vi "Parse RMC Sentence.vi"(8 "error in (no error)":errorcluster, 11 "RMC sentence":string) -> (0 "error out":errorcluster, 3 "RMC data":T1 {"type of fix"."mode" items=["", "Simulator", "Not Valid", "Estimated", "Differential", "Autonomous"]; "status"."value" items=["Void", "Active", ""]; "time of fix"."time" format="%^<%.3X\n%x>T"})   [LabVIEW 2011, in "u-blox 5 Series.lvlib"]
doc: "Returns data contained in an NMEA sentence. You must manually select the polymorphic instance to use."
uses:
  u-blox 5 Series.lvlib
  typedefs/RMC Data.ctl
  <vilib>/Utility/miscctls.llb/LVDateTimeRec.ctl
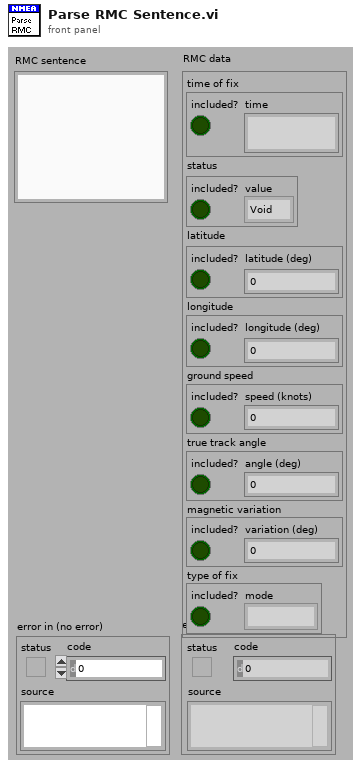
[diagram p1: front panel]
types:
  T1 = typedef "u-blox 5 Series.lvlib/RMC Data.ctl" = cluster{"time of fix":cluster{"included?":bool, "time":timestamp}, "status":cluster{"included?":bool, "value":u16}, "latitude":cluster{"included?":bool, "latitude (deg)":dbl}, "longitude":cluster{"included?":bool, "longitude (deg)":dbl}, "ground speed":cluster{"included?":bool, "speed (knots)":dbl}, "true track angle":cluster{"included?":bool, "angle (deg)":dbl}, "magnetic variation":cluster{"included?":bool, "variation (deg)":dbl}, "type of fix":cluster{"included?":bool, "mode":u16}}
  T2 = typedef "LVDateTimeRec.ctl" = cluster{"fractional second":dbl, "second":i32, "minute":i32, "hour":i32, "day of month":i32, "month":i32, "year":i32, "day of week":i32, "day of year":i32, "DST":i32}
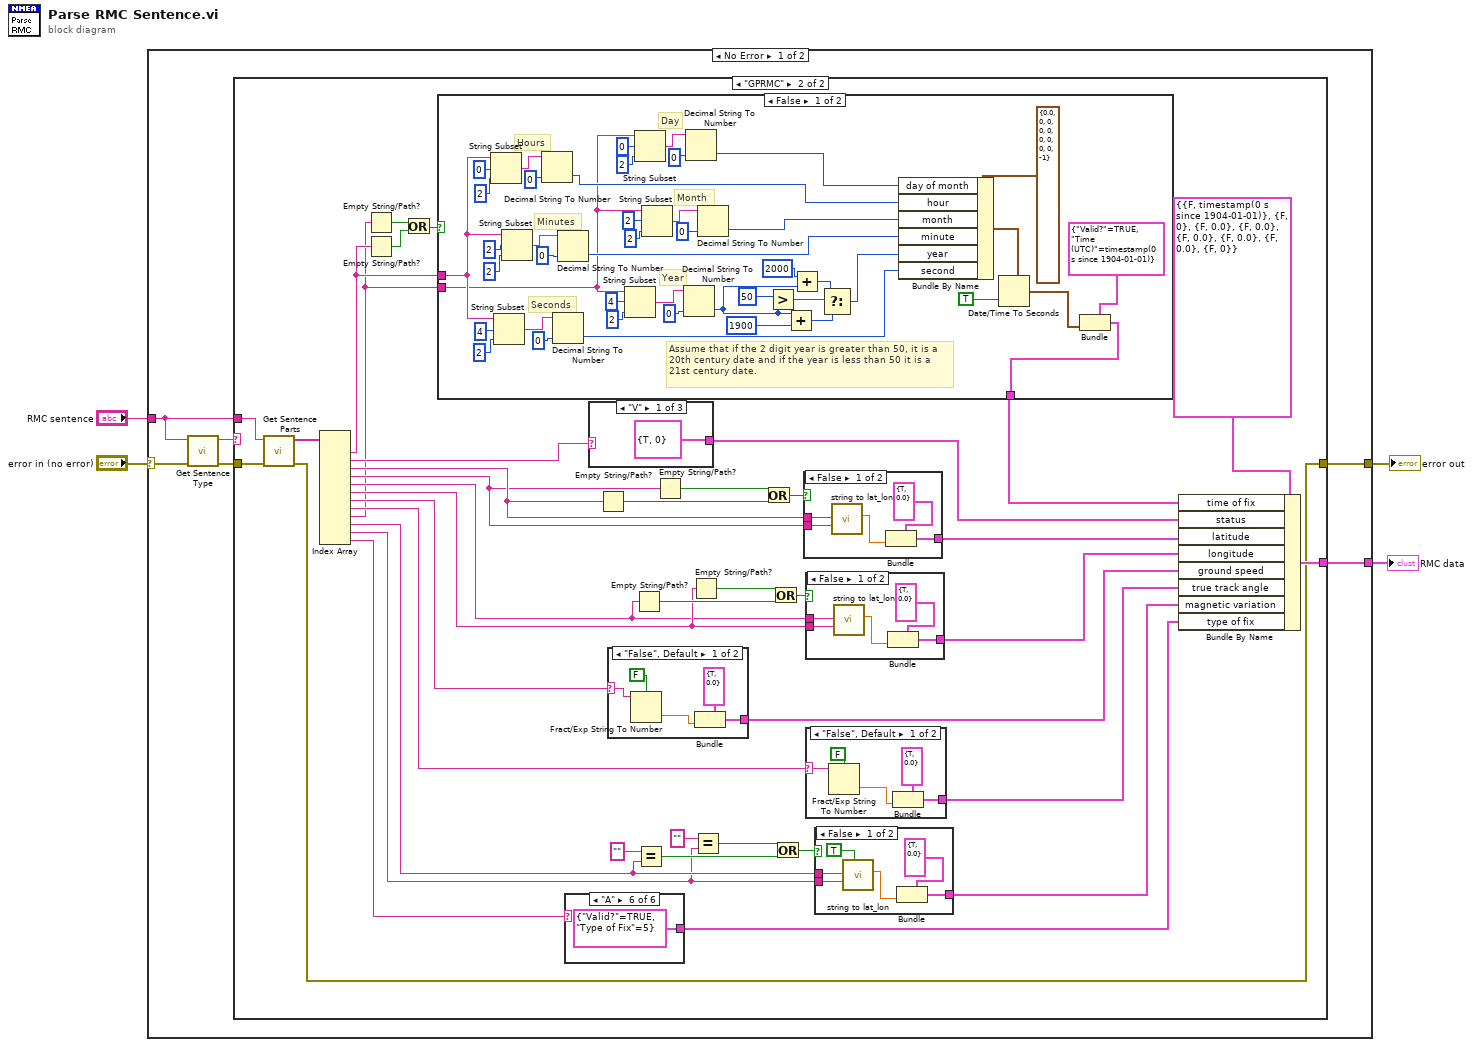
[diagram p0: block diagram]
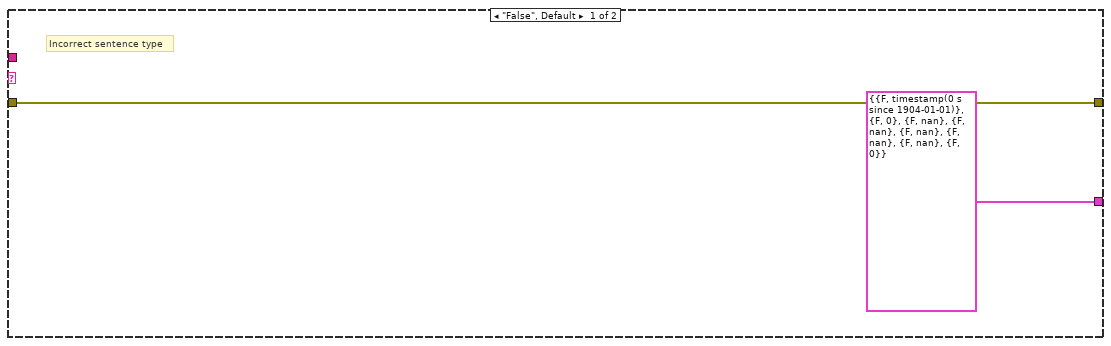
[diagram p2: hidden frame]
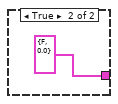
[diagram p3: hidden frame]
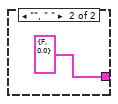
[diagram p4: hidden frame]
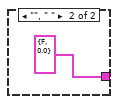
[diagram p5: hidden frame]
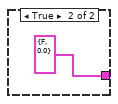
[diagram p6: hidden frame]
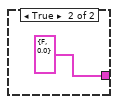
[diagram p7: hidden frame]
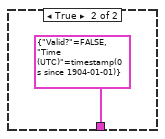
[diagram p8: hidden frame]
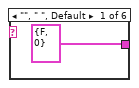
[diagram p9: hidden frame]
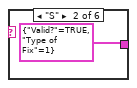
[diagram p10: hidden frame]
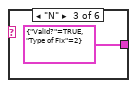
[diagram p11: hidden frame]
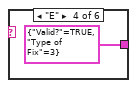
[diagram p12: hidden frame]
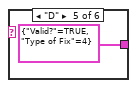
[diagram p13: hidden frame]
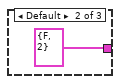
[diagram p14: hidden frame]
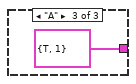
[diagram p15: hidden frame]
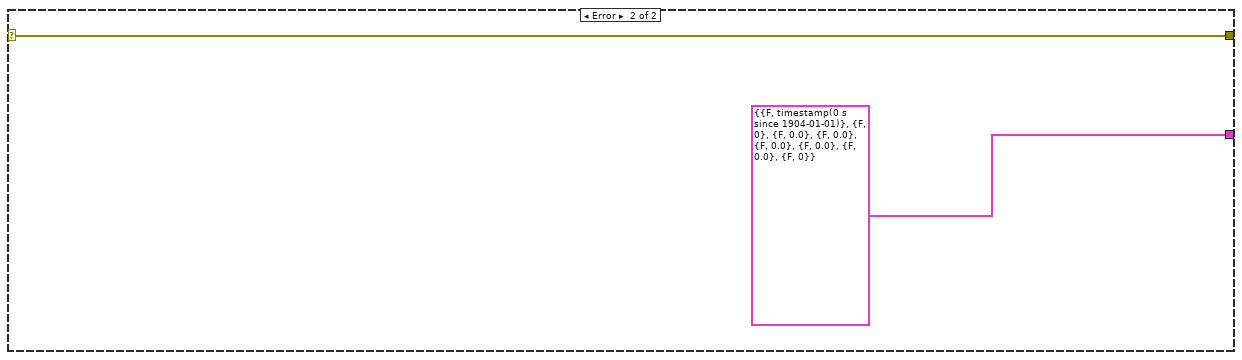
[diagram p16: hidden frame]
diagram:
  n1 = case shown="No Error" "error in (no error)" {
    selector: "error in (no error)" -> [w8 w140]
    tunnel: [w9 w140] -> w2
    tunnel: [w10 T1 {"time of fix"={"included?"=FALSE, "time"=timestamp(0 s since 1904-01-01)}, "status"={"included?"=FALSE, "value"=0}, "latitude"={"included?"=FALSE, "latitude (deg)"=0.0}, "longitude"={"included?"=FALSE, "longitude (deg)"=0.0}, "ground speed"={"included?"=FALSE, "speed (knots)"=0.0}, "true track angle"={"included?"=FALSE, "angle (deg)"=0.0}, "magnetic variation"={"included?"=FALSE, "variation (deg)"=0.0}, "type of fix"={"included?"=FALSE, "mode"=0}} ("RMC Data")] -> w1
    tunnel: "RMC sentence" -> [w6 _]
    frame No Error {
      n2 = call "Get Sentence Type.vi"("error in (no error)"=w8, "sentence"=w6) -> ("error out"=w7:errorcluster, "sentence type"=w5:string)  [unwired: 1 in, 7 out]
      n3 = case shown="\"GPRMC\"" w5 {
        tunnel: w6 -> [_ w16]
        tunnel: w7 -> [w11 w52]
        tunnel: [T1 {"time of fix"={"included?"=FALSE, "time"=timestamp(0 s since 1904-01-01)}, "status"={"included?"=FALSE, "value"=0}, "latitude"={"included?"=FALSE, "latitude (deg)"=nan}, "longitude"={"included?"=FALSE, "longitude (deg)"=nan}, "ground speed"={"included?"=FALSE, "speed (knots)"=nan}, "true track angle"={"included?"=FALSE, "angle (deg)"=nan}, "magnetic variation"={"included?"=FALSE, "variation (deg)"=nan}, "type of fix"={"included?"=FALSE, "mode"=0}} ("RMC Data") w51] -> w10
        tunnel: [w11 w14] -> w9
        frame "False", Default {
          # "Incorrect sentence type"
        }
        frame "GPRMC" {
          n4 = call "Get Sentence Parts.vi"("error in (no error)"=w52, "sentence"=w16) -> ("error out"=w14:errorcluster, "sentence data"=w15:string[])  [unwired: 1 in, 7 out]
          n5 = Index Array(array=w15) -> (element #1=w44:string, element #2=w49:string, element #3=w40:string, element #4=w39:string, element #5=w30:string, element #6=w31:string, element #7=w29:string, element #8=w27:string, element #9=w13:string, element #10=w20:string, element #11=w19:string, element #12=w48:string)  [unwired: 12 in]
          n6 = Empty String/Path?(string/path=w13) -> (empty?=w46:bool)
          n7 = Empty String/Path?(string/path=w44) -> (empty?=w47:bool)
          n8 = Or(x=w46, y=w47) -> (x .or. y?=w45:bool)
          n9 = case shown="False" w45 {
            tunnel: [w93 cluster{"Valid?":bool, "Time (UTC)":timestamp} {"Valid?"=FALSE, "Time (UTC)"=timestamp(0 s since 1904-01-01)} ("Time of Fix")] -> w43
            tunnel: w44 -> [w97 _]
            tunnel: w13 -> [w96 _]
            frame False {
              # "Assume that if the 2 digit year is greater than 50, it is a\n20th century date and if the year is less than 50 it is a \n21st century date."
              # "Year"
              # "Month"
              # "Day"
              # "Seconds"
              # "Minutes"
              # "Hours"
              n10 = String Subset(string=w97, offset (0)=0 ("length (rest)"), length (rest)=2 ("length (rest)")) -> (substring=w121:string)
              n11 = String Subset(string=w97, offset (0)=4 ("length (rest)"), length (rest)=2 ("length (rest)")) -> (substring=w125:string)
              n12 = String Subset(string=w97, offset (0)=2 ("length (rest)"), length (rest)=2 ("length (rest)")) -> (substring=w122:string)
              n13 = Decimal String To Number(string=w121, default (0L)=0 ("default (0 DBL)")) -> (number=w103:i32)  [unwired: 2 out]
              n14 = Decimal String To Number(string=w125, default (0L)=0 ("default (0 DBL)")) -> (number=w100:i32)  [unwired: 2 out]
              n15 = Decimal String To Number(string=w122, default (0L)=0 ("default (0 DBL)")) -> (number=w101:i32)  [unwired: 2 out]
              n16 = String Subset(string=w96, offset (0)=4 ("length (rest)"), length (rest)=2 ("length (rest)")) -> (substring=w114:string)
              n17 = String Subset(string=w96, offset (0)=0 ("length (rest)"), length (rest)=2 ("length (rest)")) -> (substring=w118:string)
              n18 = String Subset(string=w96, offset (0)=2 ("length (rest)"), length (rest)=2 ("length (rest)")) -> (substring=w117:string)
              n19 = Decimal String To Number(string=w114, default (0L)=0 ("default (0 DBL)")) -> (number=w87:i32)  [unwired: 2 out]
              n20 = Decimal String To Number(string=w118, default (0L)=0 ("default (0 DBL)")) -> (number=w104:i32)  [unwired: 2 out]
              n21 = Decimal String To Number(string=w117, default (0L)=0 ("default (0 DBL)")) -> (number=w102:i32)  [unwired: 2 out]
              n22 = Greater?(x=50, y=w87) -> (0:w91:bool)
              n23 = Add(x=w87, y=1900) -> (x+y=w89:i32)
              n24 = Add(x=2000, y=w87) -> (x+y=w88:i32)
              n25 = Select(t=w88, s=w91, f=w89) -> (s? t:f=w85:i32)
              n26 = Bundle By Name(cluster=T2 {"fractional second"=0.0, "second"=0, "minute"=0, "hour"=0, "day of month"=0, "month"=0, "year"=0, "day of week"=0, "day of year"=0, "DST"=-1} ("date time rec"), "day of month"=w104, "hour"=w103, "month"=w102, "minute"=w101, "year"=w85, "second"=w100) -> (w99:T2)
              n27 = Date/Time To Seconds(1:TRUE, 2:w99) -> (0:w94:timestamp)
              n28 = Bundle(cluster=cluster{"Valid?":bool, "Time (UTC)":timestamp} {"Valid?"=TRUE, "Time (UTC)"=timestamp(0 s since 1904-01-01)} ("Time of Fix"), "Time (UTC)"=w94) -> (w93:cluster{"Valid?":bool, "Time (UTC)":timestamp})  [unwired: 1 out]
            }
            frame True {
            }
          }
          n29 = case shown="\"A\"" w48 {
            tunnel: [cluster{"Valid?":bool, "Type of Fix":u16} {"Valid?"=FALSE, "Type of Fix"=0} ("Type of Fix") cluster{"Valid?":bool, "Type of Fix":u16} {"Valid?"=TRUE, "Type of Fix"=1} ("Type of Fix") cluster{"Valid?":bool, "Type of Fix":u16} {"Valid?"=TRUE, "Type of Fix"=2} ("Type of Fix") cluster{"Valid?":bool, "Type of Fix":u16} {"Valid?"=TRUE, "Type of Fix"=3} ("Type of Fix") cluster{"Valid?":bool, "Type of Fix":u16} {"Valid?"=TRUE, "Type of Fix"=4} ("Type of Fix") cluster{"Valid?":bool, "Type of Fix":u16} {"Valid?"=TRUE, "Type of Fix"=5} ("Type of Fix")] -> w17
            frame "", " ", Default {
            }
            frame "S" {
            }
            frame "N" {
            }
            frame "E" {
            }
            frame "D" {
            }
            frame "A" {
            }
          }
          n30 = case shown="\"V\"" w49 {
            tunnel: [cluster{"Valid?":bool, "Status":u16} {"Valid?"=TRUE, "Status"=0} ("Status") cluster{"Valid?":bool, "Status":u16} {"Valid?"=FALSE, "Status"=2} ("Status") cluster{"Valid?":bool, "Status":u16} {"Valid?"=TRUE, "Status"=1} ("Status")] -> w38
            frame "V" {
            }
            frame Default {
            }
            frame "A" {
            }
          }
          n31 = Empty String/Path?(string/path=w40) -> (empty?=w41:bool)
          n32 = case shown="\"False\", Default" w29 {
            selector: w29 -> [w70 _]
            tunnel: [w67 cluster{"Valid?":bool, "Speed (Knots)":dbl} {"Valid?"=FALSE, "Speed (Knots)"=0.0} ("Ground Speed")] -> w28
            frame "False", Default {
              n33 = Fract/Exp String To Number(use system decimal point (T)=FALSE, string=w70) -> (number=w68:dbl)  [unwired: 3 out]
              n34 = Bundle(cluster=cluster{"Valid?":bool, "Speed (Knots)":dbl} {"Valid?"=TRUE, "Speed (Knots)"=0.0} ("Ground Speed"), "Speed (Knots)"=w68) -> (w67:cluster{"Valid?":bool, "Speed (Knots)":dbl})  [unwired: 1 out]
            }
            frame "", " " {
            }
          }
          n35 = Empty String/Path?(string/path=w30) -> (empty?=w34:bool)
          n36 = Equal?(x="", y=w20) -> (x = y?=w22:bool)
          n37 = Empty String/Path?(string/path=w39) -> (empty?=w42:bool)
          n38 = Empty String/Path?(string/path=w31) -> (empty?=w33:bool)
          n39 = Equal?(x="", y=w19) -> (x = y?=w23:bool)
          n40 = Or(x=w42, y=w41) -> (x .or. y?=w37:bool)
          n41 = Or(x=w33, y=w34) -> (x .or. y?=w32:bool)
          n42 = Or(x=w23, y=w22) -> (x .or. y?=w21:bool)
          n43 = case shown="False" w37 {
            tunnel: w40 -> [w82 _]
            tunnel: w39 -> [w81 _]
            tunnel: [w78 cluster{"Valid?":bool, "Latitude (Deg)":dbl} {"Valid?"=FALSE, "Latitude (Deg)"=0.0} ("Latitude")] -> w36
            frame False {
              n44 = call "string to lat_lon.vi"("direction string"=w81, "numeric string for lat/lon"=w82) -> ("composite value"=w80:dbl)  [unwired: 1 in, 8 out]
              n45 = Bundle(cluster=cluster{"Valid?":bool, "Latitude (Deg)":dbl} {"Valid?"=TRUE, "Latitude (Deg)"=0.0} ("Latitude"), "Latitude (Deg)"=w80) -> (w78:cluster{"Valid?":bool, "Latitude (Deg)":dbl})  [unwired: 1 out]
            }
            frame True {
            }
          }
          n46 = case shown="False" w32 {
            tunnel: w30 -> [w76 _]
            tunnel: w31 -> [w75 _]
            tunnel: [w72 cluster{"Valid?":bool, "Latitude (Deg)":dbl} {"Valid?"=FALSE, "Latitude (Deg)"=0.0} ("Latitude")] -> w35
            frame False {
              n47 = call "string to lat_lon.vi"("direction string"=w75, "numeric string for lat/lon"=w76) -> ("composite value"=w74:dbl)  [unwired: 1 in, 8 out]
              n48 = Bundle(cluster=cluster{"Valid?":bool, "Latitude (Deg)":dbl} {"Valid?"=TRUE, "Latitude (Deg)"=0.0} ("Latitude"), "Latitude (Deg)"=w74) -> (w72:cluster{"Valid?":bool, "Latitude (Deg)":dbl})  [unwired: 1 out]
            }
            frame True {
            }
          }
          n49 = case shown="\"False\", Default" w27 {
            selector: w27 -> [w64 _]
            tunnel: [w61 cluster{"Valid?":bool, "Speed (Knots)":dbl} {"Valid?"=FALSE, "Speed (Knots)"=0.0} ("Ground Speed")] -> w26
            frame "False", Default {
              n50 = Fract/Exp String To Number(use system decimal point (T)=FALSE, string=w64) -> (number=w62:dbl)  [unwired: 3 out]
              n51 = Bundle(cluster=cluster{"Valid?":bool, "Speed (Knots)":dbl} {"Valid?"=TRUE, "Speed (Knots)"=0.0} ("Ground Speed"), "Speed (Knots)"=w62) -> (w61:cluster{"Valid?":bool, "Speed (Knots)":dbl})  [unwired: 1 out]
            }
            frame "", " " {
            }
          }
          n52 = case shown="False" w21 {
            tunnel: w20 -> [w58 _]
            tunnel: w19 -> [w57 _]
            tunnel: [w54 cluster{"Valid?":bool, "Latitude (Deg)":dbl} {"Valid?"=FALSE, "Latitude (Deg)"=0.0} ("Latitude")] -> w18
            frame False {
              n53 = call "string to lat_lon.vi"("magnetic variation?"=TRUE ("Magnetic Variation?"), "direction string"=w57, "numeric string for lat/lon"=w58) -> ("composite value"=w56:dbl)  [unwired: 8 out]
              n54 = Bundle(cluster=cluster{"Valid?":bool, "Latitude (Deg)":dbl} {"Valid?"=TRUE, "Latitude (Deg)"=0.0} ("Latitude"), "Latitude (Deg)"=w56) -> (w54:cluster{"Valid?":bool, "Latitude (Deg)":dbl})  [unwired: 1 out]
            }
            frame True {
            }
          }
          n55 = Bundle By Name(cluster=T1 {"time of fix"={"included?"=FALSE, "time"=timestamp(0 s since 1904-01-01)}, "status"={"included?"=FALSE, "value"=0}, "latitude"={"included?"=FALSE, "latitude (deg)"=0.0}, "longitude"={"included?"=FALSE, "longitude (deg)"=0.0}, "ground speed"={"included?"=FALSE, "speed (knots)"=0.0}, "true track angle"={"included?"=FALSE, "angle (deg)"=0.0}, "magnetic variation"={"included?"=FALSE, "variation (deg)"=0.0}, "type of fix"={"included?"=FALSE, "mode"=0}} ("RMC Data"), "time of fix"=w43, "status"=w38, "latitude"=w36, "longitude"=w35, "ground speed"=w28, "true track angle"=w26, "magnetic variation"=w18, "type of fix"=w17) -> (w51:T1)
        }
      }
    }
    frame Error {
    }
  }
  "error out" <- w2
  "RMC data" <- w1
